vi "LVProjectShortcut_Item_OnWizardComplete.vi"(11 "Object":T1) -> ()   [LabVIEW 2017]
doc: "Notifies the project item that the Create New Wizard process is finished."
uses:
  <resource>/Framework/Providers/API/ItemRef.ctl
panel:
  out "error out":errorcluster
  in  "error in":errorcluster
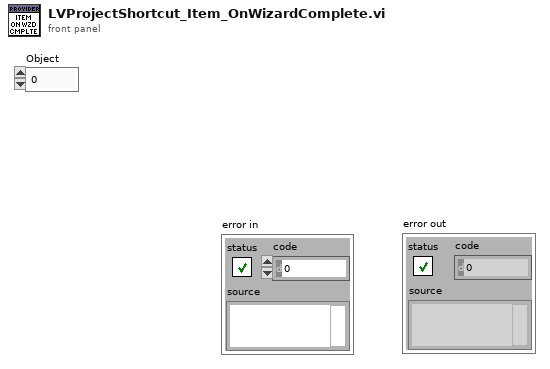
[diagram p1: front panel]
types:
  T1 = typedef "ItemRef.ctl" = u64
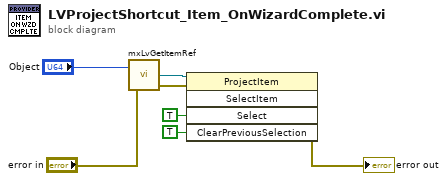
[diagram p0: block diagram]
diagram:
  n1 = call <resource>:"mxLvGetItemRef.vi"("Item"="Object", "error in"="error in") -> ("Item Refnum"=w6:refnum<vi>, "error out"=w5:errorcluster)  [unwired: 1 out]
  n2 = invoke class="ProjectItem" method="SelectItem"(reference=w6, error in=w5, "Select"=TRUE, "ClearPreviousSelection"=TRUE) -> (error out=→"error out":errorcluster)  [unwired: 1 in, 4 out]
